vi "XImc simple example with network.vi"() -> ()   [LabVIEW 2012]
uses:
  libximc.lvlib
panel:
  in  "error in (no error)":errorcluster
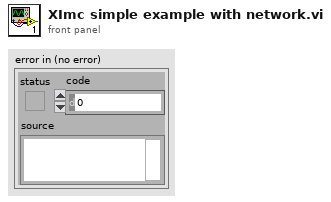
[diagram p1: front panel]
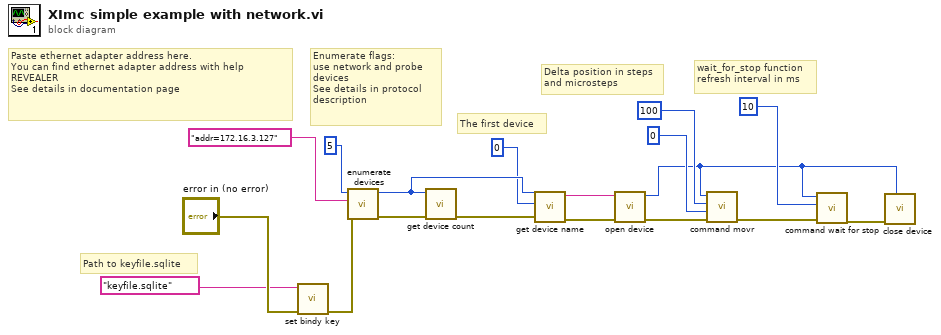
[diagram p0: block diagram]
diagram:
  # "Enumerate flags:\nuse network and probe devices\nSee details in protocol description"
  # "The first device"
  # "Path to keyfile.sqlite"
  # "Paste ethernet adapter address here.\nYou can find ethernet adapter address with help REVEALER\nSee details in documentation page"
  # "Delta position in steps and microsteps"
  # "wait_for_stop function refresh interval in ms"
  n1 = call "set bindy key.vi"("error in (no error)"="error in (no error)", "keyfilepath"="keyfile.sqlite") -> ("error out"=w3:errorcluster)  [unwired: 8 in, 1 out]
  n2 = call "enumerate devices.vi"("error in (no error)"=w3, "hints"="addr=172.16.3.127", "enumerate_flags"=5 ("probe_devices")) -> ("error out"=w17:errorcluster, "function return"=w15:u64)  [unwired: 7 in]
  n3 = call "get device count.vi"("error in (no error)"=w17, "device_enumeration"=w15) -> ("error out"=w16:errorcluster)  [unwired: 8 in, 1 out]
  n4 = call "get device name.vi"("error in (no error)"=w16, "device_index"=0 ("probe_devices"), "device_enumeration"=w15) -> ("error out"=w12:errorcluster, "function return"=w13:string)  [unwired: 7 in]
  n5 = call "open device.vi"("error in (no error)"=w12, "name"=w13) -> ("error out"=w10:errorcluster, "function return"=w5:i32)  [unwired: 8 in]
  n6 = call "command movr.vi"("error in (no error)"=w10, "uDeltaPosition"=0 ("probe_devices"), "DeltaPosition"=100 ("probe_devices"), "id"=w5) -> ("error out"=w9:errorcluster)  [unwired: 6 in, 1 out]
  n7 = call "command wait for stop.vi"("error in (no error)"=w9, "refresh_interval_ms"=10 ("probe_devices"), "id"=w5) -> ("error out"=w7:errorcluster)  [unwired: 7 in, 1 out]
  n8 = call "close device.vi"("error in (no error)"=w7, "id"=w5) -> ()  [unwired: 7 in, 3 out]
